vi "csm-lv-project.vi"() -> ()   [LabVIEW 2017, in "testcase-documentation.lvclass"]
uses:
  testcase-documentation.lvclass
  src/project/Communicable State Machine(CSM)/csm_tool_menu.lvlib
panel:
  out "error out":errorcluster
  in  "error in (no error)":errorcluster
  in  "VI Ref":refnum<vi>
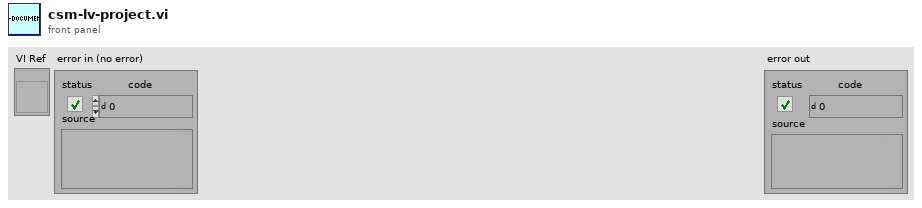
[diagram p1: front panel]
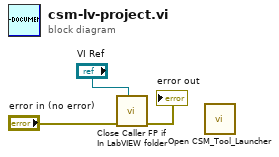
[diagram p0: block diagram]
diagram:
  n1 = call "Close Caller FP if In LabVIEW folder.vi"("VI Ref"="VI Ref", "error in (no error)"="error in (no error)") -> ("error out"=→"error out":errorcluster)  [unwired: 9 in]
  n2 = call "Open CSM_Tool_Launcher.vi"() -> ()  [unwired: 12 in]
